vi "Write.vi"(8 "error in (no error)":errorcluster, 10 "Interface":refnum<class "Interface.lvclass">, 11 "Section in":refnum<class "Section.lvclass">) -> (0 "error out":errorcluster, 3 "Section out":refnum<class "Section.lvclass">)   [LabVIEW 2013, in "Configuration.lvlib" / "Section.lvclass"]
doc: "Write section data to interface.\n\n<b>Channeling Pattern:</b> This public methode calls the protected method <b>Do Write.vi</b> overwritten by child classes. Some pre- or post-processing can be implemented here and garanteed."
uses:
  Section.lvclass
  Interface/Interface.lvclass
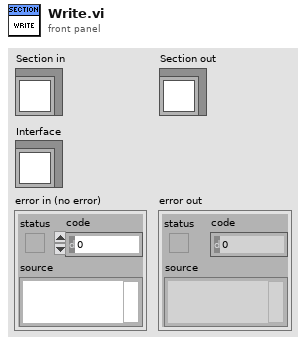
[diagram p1: front panel]
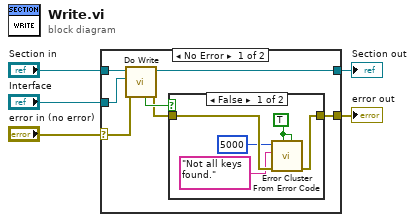
[diagram p0: block diagram]
diagram:
  n1 = case shown="No Error" "error in (no error)" {
    selector: "error in (no error)" -> [w10 w20]
    tunnel: [w7 w20] -> w4
    tunnel: [w11 w19] -> w2
    tunnel: "Section in" -> [w12 w19]
    tunnel: "Interface" -> [w6 _]
    frame No Error {
      n2 = call-dynamic "Do Write.vi"("error in (no error)"=w10, "Interface"=w6, "Section in"=w12) -> ("error out"=w8:errorcluster, "Section out"=w11:refnum<class "Section.lvclass">, "All Keys Found?"=w9:bool)  [unwired: 6 in]
      n3 = case shown="False" w9 {
        tunnel: [w16 w18] -> w7
        tunnel: w8 -> [w17 w18]
        frame False {
          w15 = TRUE ("show call chain? (False)")
          n4 = call <vilib>:"Error Cluster From Error Code.vi"("is warning? (False)"=w15, "show call chain? (False)"=w15, "error in (no error)"=w17, "error message (\"\")"="Not all keys found." ("error message (\"\")"), "error code (0)"=5000) -> ("error out"=w16:errorcluster)  [unwired: 4 in]
        }
        frame True {
        }
      }
    }
    frame Error {
    }
  }
  "error out" <- w4
  "Section out" <- w2
